vi "LoadControlPanel.vi"(8 "error in (no error)":errorcluster, 10 "Actor In":refnum<class "Actor.lvclass">, 11 "QuickNote in":refnum<class "QuickNote.lvclass">) -> (0 "error out":errorcluster, 3 "QuickNote out":refnum<class "QuickNote.lvclass">)   [LabVIEW 2020, in "QuickNote.lvlib" / "QuickNote.lvclass"]
uses:
  QuickNote.lvclass
  QuickNoteUI/QuickNoteUI.lvclass
  Hardware Abstraction Layer/Component/Device/Device/DataExchange.ctl
  Interface/DataListener/DataListener.lvclass
  Hardware Abstraction Layer/Component/GenericActor/GenericActor/GenericController.lvclass
  C:/Program Files/National Instruments/LabVIEW 2020/vi.lib/ActorFramework/Actor/Actor.lvclass
  <vilib>/ActorFramework/Actor/Actor.lvclass
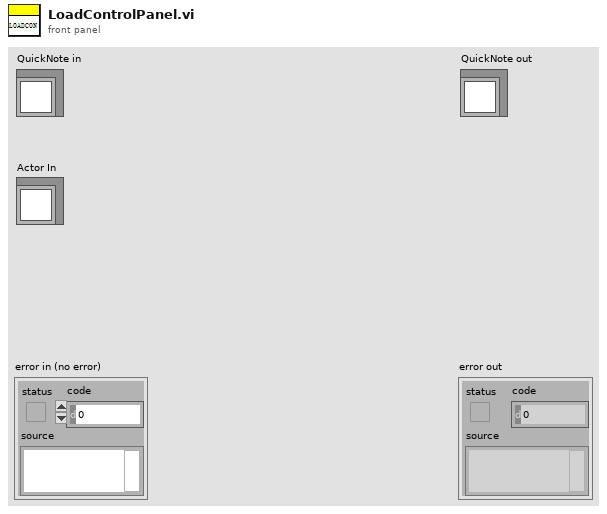
[diagram p1: front panel]
types:
  T1 = typedef "DataListener.lvclass/DataExchange.ctl" = cluster{"Source":string, "Destination":string, "Description":string, "value":variant}
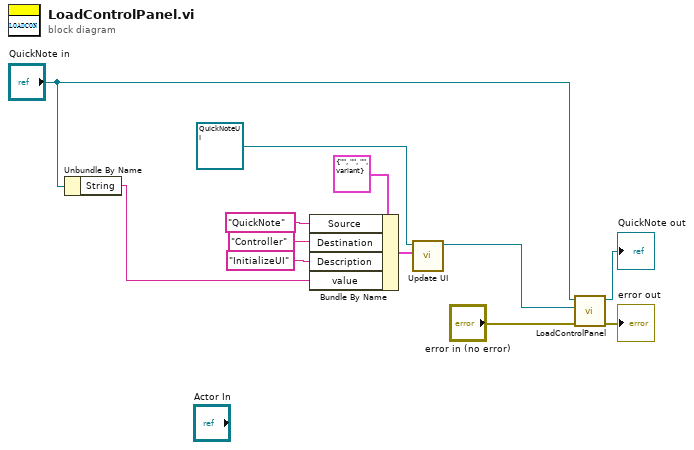
[diagram p0: block diagram]
diagram:
  n1 = Unbundle By Name("QuickNote in") -> ("String"=w3:string)
  n2 = Bundle By Name(cluster=T1 {"Source"="", "Destination"="", "Description"="", "value"=variant} ("DataExchange"), "Source"="QuickNote", "Destination"="Controller", "Description"="InitializeUI", "value"=w3) -> (w6:T1)
  n3 = call-dynamic "Update UI.vi"("DataExchange"=w6, "Controller Template in"=refnum<class "QuickNoteUI.lvclass"> refnum ("QuickNote.lvlib:QuickNoteUI.lvlib:QuickNoteUI.lvclass")) -> ("Controller Template out"=w1:refnum<class "QuickNoteUI.lvclass">)  [unwired: 8 in, 1 out]
  n4 = call-parent "LoadControlPanel.vi"("error in (no error)"="error in (no error)", "Actor In"=w1, "GRMActor in"="QuickNote in") -> ("error out"=→"error out":errorcluster, "GRMActor out"=→"QuickNote out":refnum<class "QuickNote.lvclass">)  [unwired: 7 in]
